vi "ControlServo.vi"() -> ()   [LabVIEW 2017]
uses:
  <vilib>/myRIO/Common/Instrument Driver Framework/myRIO v1.0/UART/vis/myRIO v1.0 Close UART.vi
  <vilib>/myRIO/Common/Instrument Driver Framework/Utilities/vis/FPGA Ref Manager.vi
  <vilib>/myRIO/Common/Instrument Driver Framework/myRIO v1.0/myRIO v1.0 Reset FPGA.vi
  <vilib>/myRIO/Common/Instrument Driver Framework/myRIO v1.0/IRQ/vis/myRIO v1.0 IRQ Info FGV.vi
  <vilib>/myRIO/Common/Instrument Driver Framework/myRIO v1.0/IRQ/vis/myRIO v1.0 Timer IRQ Info FGV.vi
  <vilib>/myRIO/Common/Instrument Driver Framework/myRIO v1.0/IRQ/vis/myRIO v1.0 ISR Agent.vi
  <vilib>/myRIO/Instrument Drivers/Utilities/Utilities.lvlib
panel:
  in  "Select Channel":string(combo)="Servo 1"
  in  "stop":bool
  in  "Set Servo Position (0 - 180 degrees)":u8(slide)=90 scale=0.0..180.0
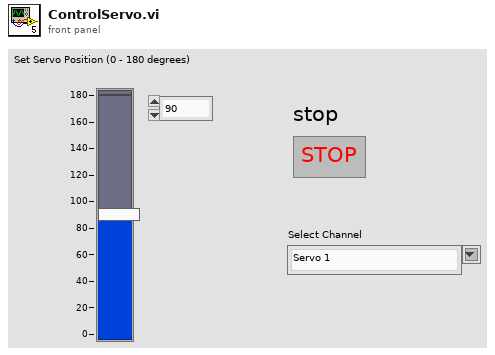
[diagram p1: front panel]
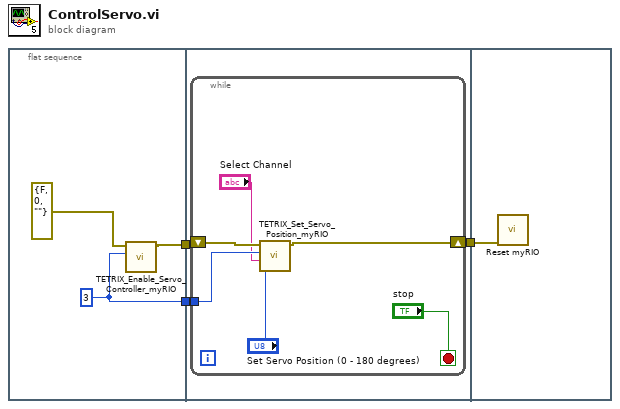
[diagram p0: block diagram]
diagram:
  n1 = flat-sequence {
    tunnel: [w5] -> w3
    tunnel: [w4] -> w2
    tunnel: w3 -> [w9]
    tunnel: w2 -> [w8]
    tunnel: [w7] -> w1
    tunnel: w1 -> [w16]
    frame #0 {
      w4 = u8 3 ("Controller ID#  (I2C Address)")
      n2 = call <vilib>:"TETRIX_Enable_Servo_Controller_myRIO.vi"("Controller ID#  (I2C Address)"=w4, "Error/Flow In"=errorcluster {"status"=FALSE, "code"=0, "source"=""} ("error constant")) -> ("Error/Flow Out"=w5:errorcluster)  [unwired: 5 in]
    }
    frame #1 {
      n3 = while {
        tunnel: w8 -> [w14]
        shift-right: [w12] -> w7
        shift-left: w9 -> [w15]
        stop <- "stop" stop-if-true
        n4 = call <vilib>:"TETRIX_Set_Servo_Position_myRIO.vi"("Set Servo Position (0 - 180 degrees)"="Set Servo Position (0 - 180 degrees)", "Select Channel"="Select Channel", "Controller ID#  (I2C Address)"=w14, "Error/Flow In"=w15) -> ("Error/Flow Out"=w12:errorcluster)  [unwired: 3 in]
      }
    }
    frame #2 {
      n5 = call <vilib>:"Reset myRIO.vi"("error in (no error)"=w16) -> ()  [unwired: 10 in, 1 out]
    }
  }
